vi "_101.vi"() -> ()   [LabVIEW 2020]
panel:
  out "Numeric":i32
  out "Numeric 2":i32
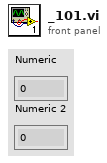
[diagram p1: front panel]
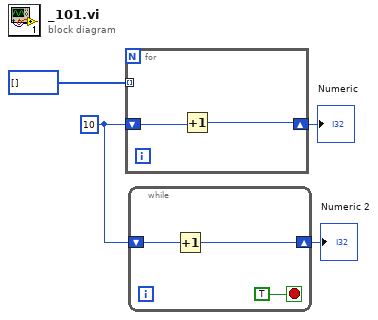
[diagram p0: block diagram]
diagram:
  w3 = 10
  n1 = for {
    tunnel: i32[] [] -> [_] mode=indexing
    shift-right: [w5] -> w1
    shift-left: w3 -> [w6]
    n2 = Increment(x=w6) -> (x+1=w5:i32)
  }
  "Numeric" <- w1
  n3 = while {
    shift-right: [w8] -> w2
    shift-left: w3 -> [w9]
    stop <- TRUE stop-if-true
    n4 = Increment(x=w9) -> (x+1=w8:i32)
  }
  "Numeric 2" <- w2
